vi "Read RC parameters_UI.vi"(0 "JSON FilePath":path=path "F:/User Interface Testbench/Configuration file/Rack Controller Override JSON UI.json", 1 "ListBox Cluster":T1, 5 "Rack Id":string="0", 7 "Variant":variant, 9 "Part Name":string, 11 "error in (no error)":errorcluster, 12 "Variant?":bool) -> (4 "Output Edit Tolerance cluster":T1, 6 "Error Message":string, 15 "error out":errorcluster)   [LabVIEW 2015, in "ZenGage v3.0 UI.lvclass"]
uses:
  ZenGage v3.0 UI.lvclass
  Common/Controls/RC override parameters.ctl
  Type Definitions/Edit tolerance settings/Rack Selection.ctl
  <vilib>/Utility/miscctls.llb/LVPoint32TypeDef.ctl
  Type Definitions/Edit tolerance settings/Edit Tolerance Input.ctl
  Type Definitions/Edit tolerance settings/ETL controls.ctl
panel:
  out "VCluster\n out":variant
  # "e"
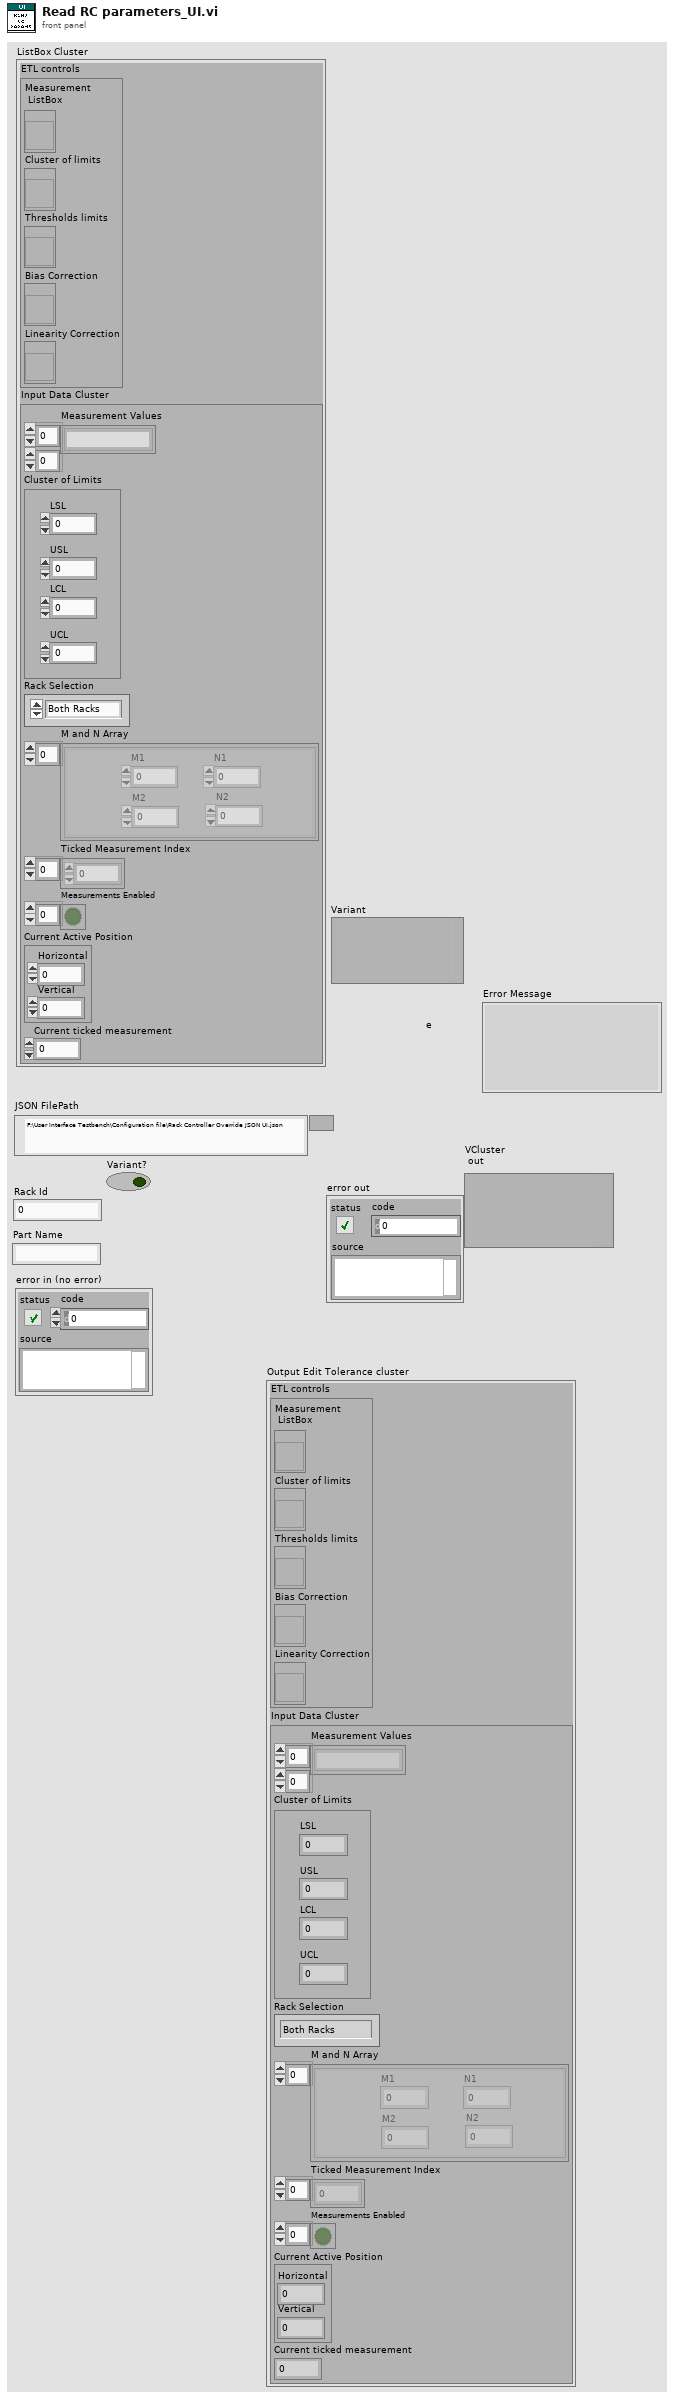
[diagram p1: front panel]
types:
  T1 = typedef "ZenGage v3.0 UI.lvclass/Edit Tolerance Input.ctl" = cluster{"ETL controls":T2, "Input Data Cluster":cluster{"Measurement Values":string[][], "Cluster of Limits":cluster{"LSL":dbl, "USL":dbl, "LCL":dbl, "UCL":dbl}, "Rack Selection":T3, "M and N Array":cluster{"M1":u64, "M2":u64, "N1":u64, "N2":u64}[], "Ticked Measurement Index":u32[], "Measurements Enabled":bool[], "Current Active Position":T4, "Current ticked measurement":dbl}}
  T2 = typedef "ETL controls.ctl" = cluster{"Measurement\n ListBox":refnum<vi>, "Cluster of limits":refnum<vi>, "Thresholds limits":refnum<vi>, "Bias Correction":refnum<vi>, "Linearity Correction":refnum<vi>}
  T3 = typedef "ZenGage v3.0 UI.lvclass/Rack Selection.ctl" = enum16{"Both Racks", "Rack 2", "Rack 1"}
  T4 = typedef "LVPoint32TypeDef.ctl" = cluster{"Horizontal":i32, "Vertical":i32}
  T5 = typedef "RC override parameters.ctl" = cluster{cluster{"Name":string, "Measurements":cluster{"MeasurementId":dbl, "Name":string, "ControlLimitsViolationThreshold":cluster{"M1":dbl, "N1":dbl}, "SpecificationLimitViolationThreshold":cluster{"M2":dbl, "N2":dbl}}[]}}
  T6 = cluster{"Name":string, "Measurements":cluster{"MeasurementId":dbl, "Name":string, "ControlLimitsViolationThreshold":cluster{"M1":dbl, "N1":dbl}, "SpecificationLimitViolationThreshold":cluster{"M2":dbl, "N2":dbl}}[]}
  T7 = cluster{"MeasurementId":dbl, "Name":string, "ControlLimitsViolationThreshold":cluster{"M1":dbl, "N1":dbl}, "SpecificationLimitViolationThreshold":cluster{"M2":dbl, "N2":dbl}}[]
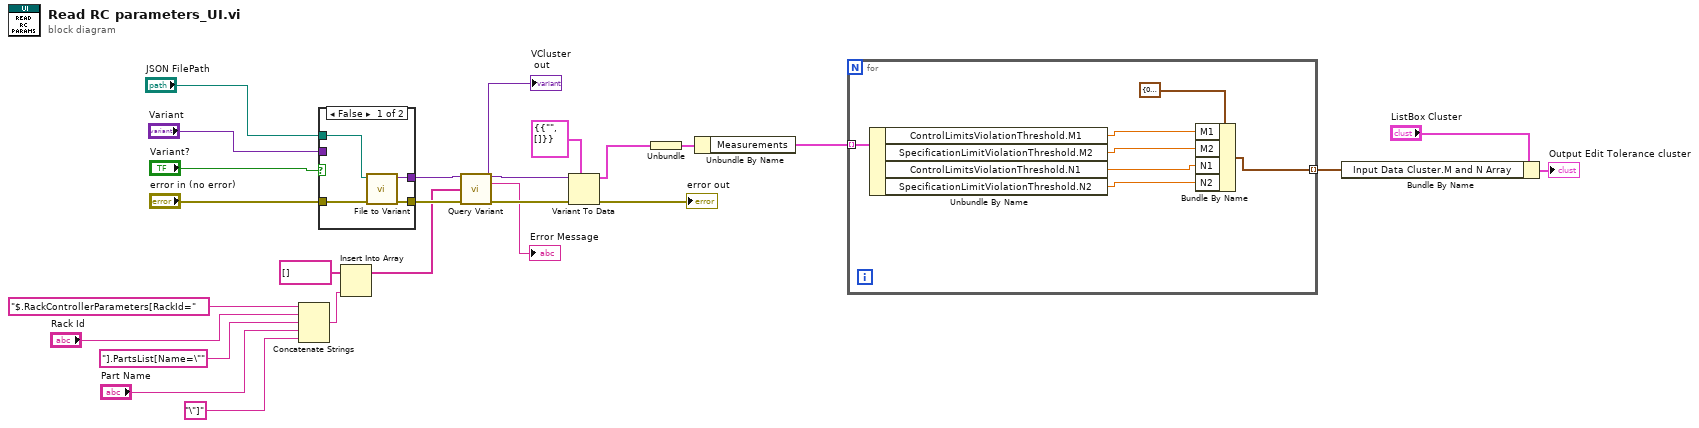
[diagram p0: block diagram]
diagram:
  n1 = Concatenate Strings("$.RackControllerParameters[RackId=" ("string"), "Rack Id", "].PartsList[Name=\"" ("string"), "Part Name", "\"]" ("string")) -> (w11:string)
  n2 = case shown="False" "Variant?" {
    tunnel: [w29 w31] -> w25
    tunnel: "error in (no error)" -> [w28 w31]
    tunnel: [w27 w30] -> w20
    tunnel: "JSON FilePath" -> [w26 _]
    tunnel: "Variant" -> [_ w30]
    frame False {
      n3 = call <vilib>:"File to Variant.vi"("JSON FilePath"=w26, "error in (no error)"=w28) -> ("JSON Variant"=w27:variant, "error out"=w29:errorcluster)  [unwired: 6 in, 1 out]
    }
    frame True {
    }
  }
  n4 = Insert Into Array(array=string[] [], new element=w11) -> (w9:string[])  [unwired: 1 in]
  n5 = call <vilib>:"Query Variant.vi"("VCluster in"=w20, "pathList"=w9, "error IO"=w25) -> ("VCluster\n out"=w21:variant, "Error Message"=→"Error Message":string, "error out"=w23:errorcluster)  [unwired: 9 in, 1 out]
  "VCluster\n out" <- w21
  n6 = Variant To Data(error in=w23, type=T5 {{"Name"="", "Measurements"=[]}}, Variant=w21) -> (data=w7:T5, error out=→"error out":errorcluster)
  n7 = Unbundle(w7) -> (w6:T6)
  n8 = Unbundle By Name(w6) -> ("Measurements"=w5:T7)
  n9 = for {
    tunnel: w5 -> [w38] mode=indexing
    tunnel: [w32] -> w4 mode=indexing
    n10 = Unbundle By Name(w38) -> ("ControlLimitsViolationThreshold.M1"=w36:dbl, "SpecificationLimitViolationThreshold.M2"=w35:dbl, "ControlLimitsViolationThreshold.N1"=w34:dbl, "SpecificationLimitViolationThreshold.N2"=w33:dbl)
    n11 = Bundle By Name(cluster=cluster{"M1":u64, "M2":u64, "N1":u64, "N2":u64} {"M1"=0, "M2"=0, "N1"=0, "N2"=0} ("Rack 1"), "M1"=w36, "M2"=w35, "N1"=w34, "N2"=w33) -> (w32:cluster{"M1":u64, "M2":u64, "N1":u64, "N2":u64})
  }
  n12 = Bundle By Name(cluster="ListBox Cluster", "Input Data Cluster.M and N Array"=w4) -> (→"Output Edit Tolerance cluster":T1)
